vi "Read SV Container.vi"(8 "error in (no error)":errorcluster, 11 "SharedVariable_Bus in":refnum<class "SharedVariable_Bus.lvclass">) -> (0 "error out":errorcluster, 2 "SV Container":refnum<k21>, 3 "SharedVariable_Bus out":refnum<class "SharedVariable_Bus.lvclass">)   [LabVIEW 2021, in "SharedVariable_Bus.lvclass"]
uses:
  SharedVariable_Bus.lvclass
  SharedVariable_Bus.lvclass/SharedVariable_Bus.ctl
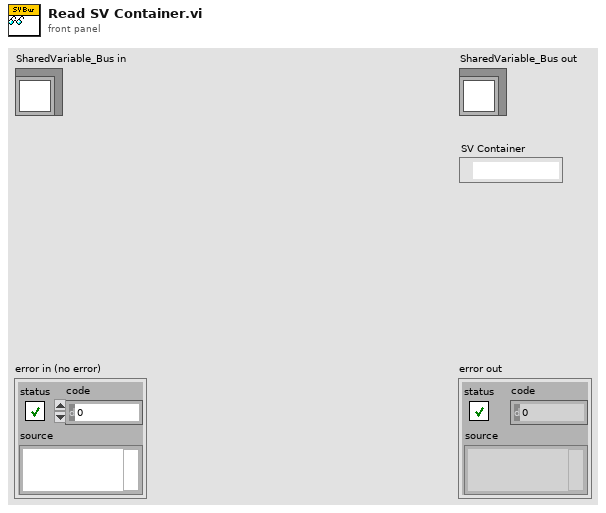
[diagram p1: front panel]
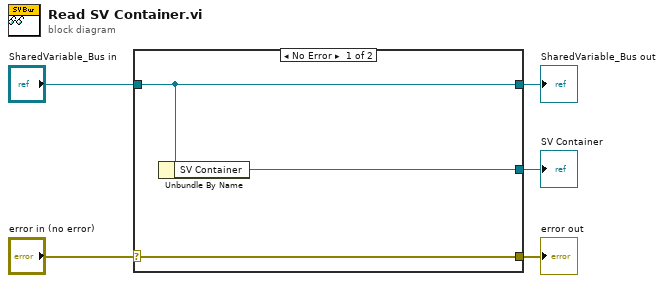
[diagram p0: block diagram]
diagram:
  n1 = case shown="No Error" "error in (no error)" {
    selector: "error in (no error)" -> [w8 w9]
    tunnel: [w8 w9] -> w4
    tunnel: [w7 w10] -> w2
    tunnel: "SharedVariable_Bus in" -> [w7 w10]
    tunnel: [w6 _] -> w1
    frame No Error {
      n2 = Unbundle By Name(w7) -> ("SV Container"=w6:refnum<k21>)
    }
    frame Error {
    }
  }
  "error out" <- w4
  "SharedVariable_Bus out" <- w2
  "SV Container" <- w1
